vi "SL1.vi"   [LabVIEW 2014, in "Lego_Swerve_2015.lvrbt"]
uses:
  Lego_Swerve_2015.lvrbt
  <vilib>/NXT/Dual Mode Library/BT/BlueTooth_Read_string.vi
  <vilib>/NXT/Dual Mode Library/Display/drawText.vi
types:
  T1 = typedef "LVHSConnector.ctl" = refnum<class "BrickReference.lvclass">
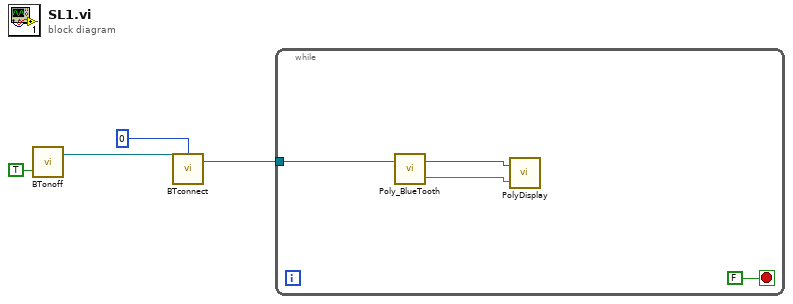
[diagram p0: block diagram]
diagram:
  n1 = call <vilib>:"BTonoff.vi"("On/Off"=TRUE) -> ("NXT/EV3"=w4:T1)  [unwired: 2 in, 1 out]
  n2 = call <vilib>:"BTconnect.vi"("NXT/EV3"=w4, "Connection"=u8 0) -> ("NXT/EV3"=w2:T1)  [unwired: 1 in, 1 out]
  n3 = while {
    tunnel: w2 -> [w7]
    stop <- FALSE stop-if-true
    n4 = call-poly <vilib>:"Poly_BlueTooth.vi"("NXT/EV3"=w7) -> ("Message"=w5:string, "NXT/EV3"=w6:T1)  [unwired: 2 in]
    n5 = call-poly <vilib>:"PolyDisplay.vi"("Text"=w5, "NXT/EV3"=w6) -> ()  [unwired: 2 in, 1 out]
  }
